vi "格式化输出.vi"(8 "错误输入（无错误）":errorcluster, 10 "字符串引用":refnum<vi>, 11 "字符串":string) -> (3 "错误输出":errorcluster)   [LabVIEW 2011]
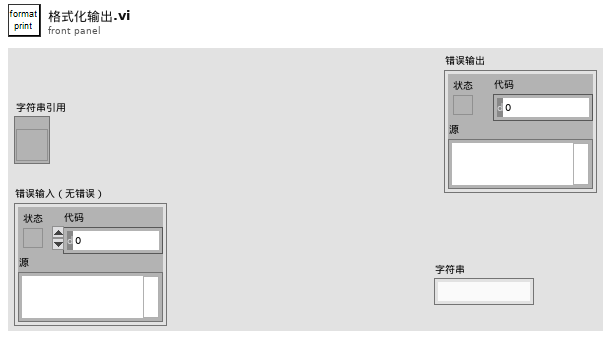
[diagram p1: front panel]
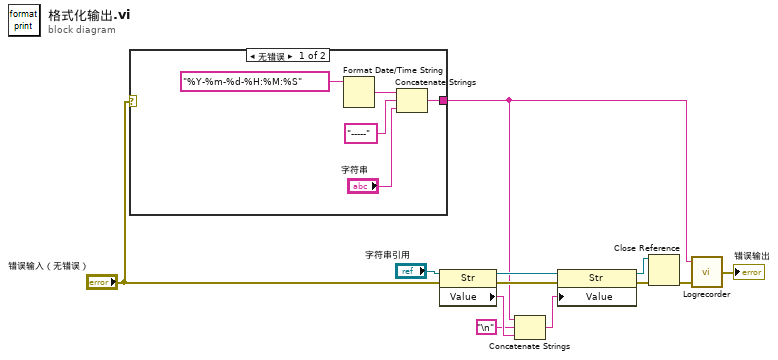
[diagram p0: block diagram]
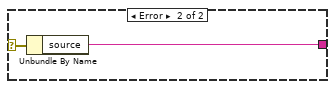
[diagram p2: hidden frame]
diagram:
  n1 = case shown="无错误" "错误输入（无错误）" {
    selector: "错误输入（无错误）" -> [_ w19]
    tunnel: [w13 w18] -> w1
    frame No Error {
      n2 = Format Date/Time String(time format string (%c)="%Y-%m-%d-%H:%M:%S" ("时间格式字符串(%c)")) -> (date/time string=w14:string)  [unwired: 2 in]
      n3 = Concatenate Strings(w14, "-----" ("字符串"), "字符串") -> (w13:string)
    }
    frame Error {
      n4 = Unbundle By Name(w19) -> ("source"=w18:string)
    }
  }
  n5 = property class="Str"(reference="字符串引用", error in="错误输入（无错误）") -> (reference out=w7:refnum<vi>, error out=w6:errorcluster, "Value"=w11:string)
  n6 = Concatenate Strings(w1, "\n", w11) -> (w5:string)
  n7 = property class="Str"(reference=w7, error in=w6, "Value"=w5) -> (reference out=w9:refnum<vi>, error out=w8:errorcluster)
  n8 = Close Reference(reference=w9, error in (no error)=w8) -> (error out=w4:errorcluster)
  n9 = call "Logrecorder.vi"("error in"=w4, "Msg"=w1) -> ("error out"=→"错误输出":errorcluster)  [unwired: 1 in]
